vi "Autonomous Independent.vi"() -> ()   [LabVIEW 2017]
doc: "This VI is called when autonomous begins, and will automatically be terminated when autonomous ends. You can carry out timed or sensor driven robot movement independently without needing to return to the caller."
uses:
  <vilib>/Rock Robotics/WPI/Utilities/WPI_GetSetVariantRefNum.vi
  <vilib>/Rock Robotics/Network Tables/NT Read String.vi
  <vilib>/Rock Robotics/WPI/RobotDrive/WPI_RobotDriveArcadeDrive_Standard(NoSaturation).vi
  <vilib>/Rock Robotics/Network Tables/NT Write Numeric Array.vi
panel:
  out "Current Movement, for debugging":T1 {"Y Joystick Value" scale=1.0..-1.0; "X Joystick Value" scale=-1.0..1.0}
  in  "Array of robot movements":T2(array[cluster])=[{"X Joystick Value"=0.39393939393939403, "Y Joystick Value"=0.0, "Delay (sec)"=1.0, "Movement Name"="turn"}, {"X Joystick Value"=-0.3737373737373737, "Y Joystick Value"=0.0, "Delay (sec)"=1.0, "Movement Name"="turn back"}] {"Y Joystick Value" scale=1.0..-1.0; "X Joystick Value" scale=-1.0..1.0}
  # "Be sure to right-click and choose Data Operations>>Make Current Value default if you want to save the array values with the VI"
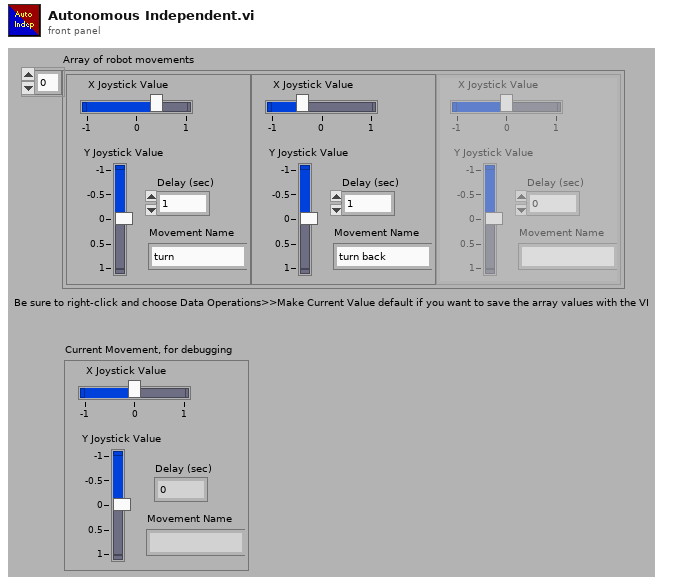
[diagram p1: front panel]
types:
  T1 = cluster{"X Joystick Value":dbl, "Y Joystick Value":dbl, "Delay (sec)":dbl, "Movement Name":string}
  T2 = cluster{"X Joystick Value":dbl, "Y Joystick Value":dbl, "Delay (sec)":dbl, "Movement Name":string}[]
  T3 = typedef "WPI_JoystickDevRef.ctl" = cluster{"Device":T4}
  T4 = typedef "WPI_JoystickDeviceEnum.ctl" = enum16{"USB 0", "USB 1", "USB 2", "USB 3", "USB 4", "USB 5"}
  T5 = typedef "WPI_RobotDriveDevRef.ctl" = cluster{"DevStatus":errorcluster, "Motors[]":T6[], "Square Inputs":bool, "Max Output":dbl}
  T6 = typedef "WPI_MotorControlDeviceRef.ctl" = cluster{"DeviceStatus":errorcluster, "Type":T7, "PWM":cluster{"PWM Channel":T8, "DeadBand":T9}, "CAN":cluster{"Device Number":u8, "SetOutput VI Ref":variant, "GetOutput VI Ref":variant, "Enable VI Ref":variant, "Disable VI Ref":variant, "Data":variant}, "Invert":bool, "DIO PWM":cluster{"PWM \"Enable\" Channel":T8, "DIOChannel":T10, "PWM Rate":dbl}}
  T7 = typedef "WPI_MotorControlType.ctl" = enum16{"PWM", "CAN", "DIO PWM"}
  T8 = typedef "FPGA_DIOPWMChannel.ctl" = enum8{"PWM 0", "PWM 1", "PWM 2", "PWM 3", "PWM 4", "PWM 5", "PWM 6", "PWM 7", "PWM 8", "PWM 9", "PWM MXP 0", "PWM MXP 1", "PWM MXP 2", "PWM MXP 3", "PWM MXP 4", "PWM MXP 5", "PWM MXP 6", "PWM MXP 7", "PWM MXP 8", "PWM MXP 9", "Invalid"}
  T9 = typedef "WPI_PWMDeadband.ctl" = cluster{"Name":string, "maxPositivePwm":i32, "minPositivePwm":i32, "centerPwm":i32, "maxNegativePwm":i32, "minNegativePwm":i32, "angularRange":u16}
  T10 = typedef "FPGA_DIOChannel.ctl" = enum8{"DIO 0", "DIO 1", "DIO 2", "DIO 3", "DIO 4", "DIO 5", "DIO 6", "DIO 7", "DIO 8", "DIO 9", "DIO MXP 0", "DIO MXP 1", "DIO MXP 2", "DIO MXP 3", "DIO MXP 4", "DIO MXP 5", "DIO MXP 6", "DIO MXP 7", "DIO MXP 8", "DIO MXP 9", "DIO MXP 10", "DIO MXP 11", "DIO MXP 12", "DIO MXP 13", "DIO MXP 14", "DIO MXP 15", "SPI Port CS1", "SPI Port CS2", "SPI Port CS3", "SPI Port MISO", "SPI Port MOSI", "Invalid"}
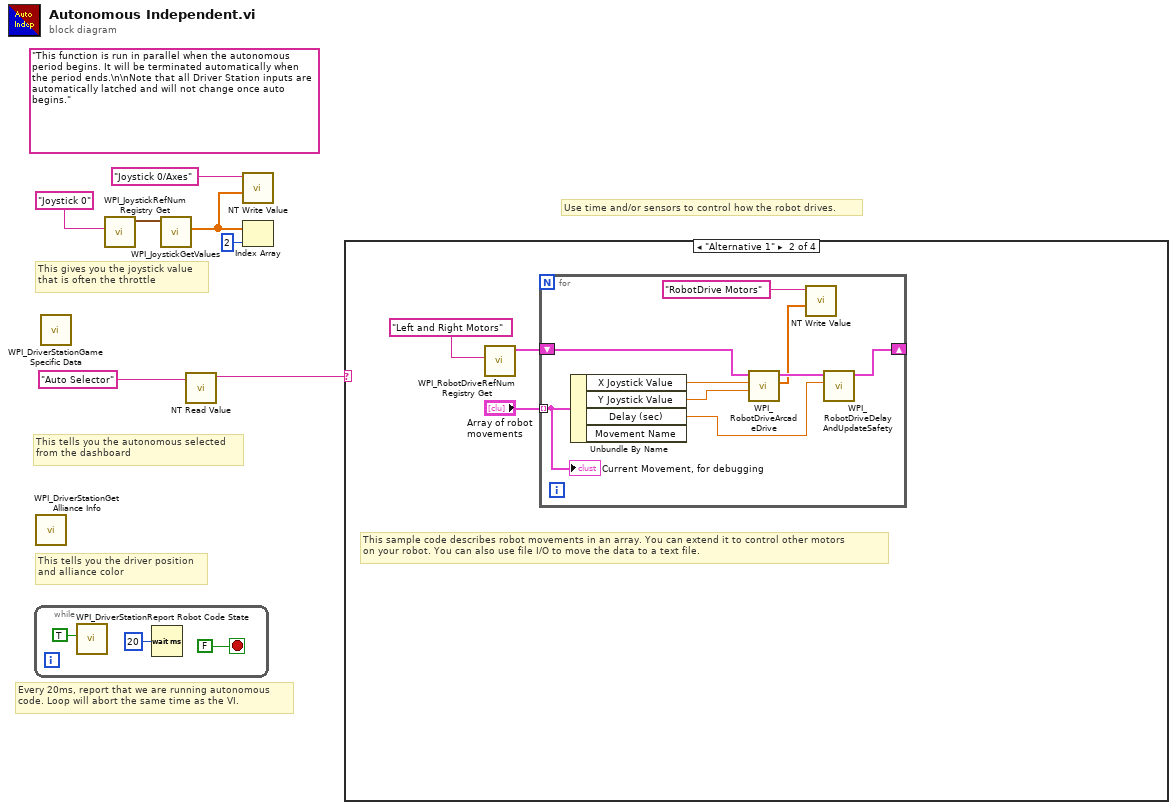
[diagram p0: block diagram]
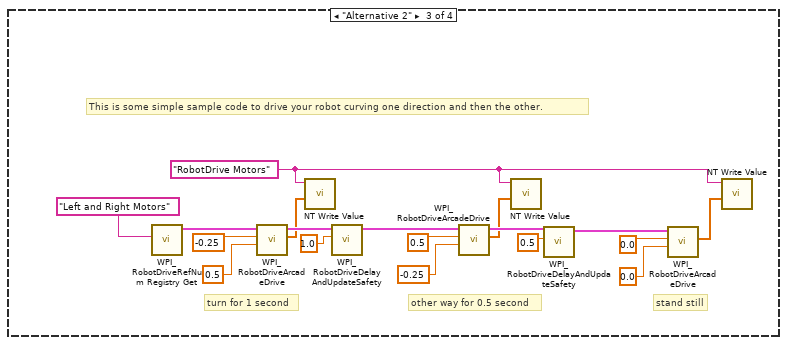
[diagram p3: hidden frame]
diagram:
  (unwired) "This function is run in parallel when the autonomous period begins. It will be terminated automatically when the period ends.\n\nNote that all Driver Station inputs are automatically latched and will not change once auto begins."
  # "This tells you the autonomous selected\nfrom the dashboard"
  # "Every 20ms, report that we are running autonomous\ncode. Loop will abort the same time as the VI."
  # "This gives you the joystick value\nthat is often the throttle"
  # "Use time and/or sensors to control how the robot drives."
  # "This tells you the driver position\nand alliance color"
  n1 = while {
    stop <- FALSE stop-if-true
    n2 = call <vilib>:"WPI_DriverStationReport Robot Code State.vi"("Autonomous"=TRUE) -> ()  [unwired: 10 in, 1 out]
    n3 = Wait (ms)(milliseconds to wait=u32 20) -> ()  [unwired: 1 out]
  }
  n4 = call <vilib>:"WPI_DriverStationGet Alliance Info.vi"() -> ()  [unwired: 12 out]
  n5 = call <vilib>:"WPI_DriverStationGame Specific Data.vi"() -> ()  [unwired: 11 in, 1 out]
  n6 = call <vilib>:"WPI_JoystickRefNum Registry Get.vi"("refnum name"="Joystick 0") -> ("JoystickDevRef"=w6:T3)  [unwired: 1 in, 9 out]
  n7 = call <vilib>:"WPI_JoystickGetValues.vi"("JoystickDevRef"=w6) -> ("Axes"=w2:dbl[])  [unwired: 6 in, 4 out]
  n8 = call-poly <vilib>:"NT Read Value.vi"("Name"="Auto Selector") -> ("String"=w3:string)  [unwired: 9 in, 1 out]
  n9 = call-poly <vilib>:"NT Write Value.vi"("Numeric Array"=w2, "Name"="Joystick 0/Axes") -> ()  [unwired: 9 in, 1 out]
  n10 = Index Array(array=w2, index=2) -> ()  [unwired: 1 out]
  n11 = case shown="\"Alternative 1\"" w3 {
    frame Default {
      # "You can put your main auto here, or you can right-click on the case and make any\nother frame be the default case."
      # "This is the frame that will execute if no selection is made, or if it is not recognized"
    }
    frame "Alternative 1" {
      # "This sample code describes robot movements in an array. You can extend it to control other motors\non your robot. You can also use file I/O to move the data to a text file."
      n12 = call <vilib>:"WPI_RobotDriveRefNum Registry Get.vi"("refnum name"="Left and Right Motors") -> ("RobotDriveDevRef"=w12:T5)  [unwired: 1 in, 9 out]
      n13 = for {
        shift-right: [w20] -> _
        shift-left: w12 -> [w21]
        tunnel: "Array of robot movements" -> [w16] mode=indexing
        n14 = Unbundle By Name(w16) -> ("X Joystick Value"=w19:dbl, "Y Joystick Value"=w18:dbl, "Delay (sec)"=w17:dbl)  [unwired: 1 out]
        n15 = call-poly <vilib>:"WPI_RobotDriveArcadeDrive.vi"("Y axis value"=w18, "X axis value"=w19, "RobotDriveDevRef"=w21) -> ("Motor Values"=w14:dbl[], "RobotDriveDevRef"=w22:T5)  [unwired: 1 in, 6 out]
        n16 = call-poly <vilib>:"NT Write Value.vi"("Numeric Array"=w14, "Name"="RobotDrive Motors") -> ()  [unwired: 9 in, 1 out]
        n17 = call <vilib>:"WPI_RobotDriveDelayAndUpdateSafety.vi"("Delay (s)"=w17, "RobotDriveDevRef"=w22) -> ("RobotDriveDevRef 2"=w20:T5)  [unwired: 8 in, 1 out]
        "Current Movement, for debugging" <- w16
      }
    }
    frame "Alternative 2" {
      w24 = "RobotDrive Motors" ("Name")
      # "This is some simple sample code to drive your robot curving one direction and then the other."
      # "stand still"
      # "other way for 0.5 second"
      # "turn for 1 second"
      n18 = call <vilib>:"WPI_RobotDriveRefNum Registry Get.vi"("refnum name"="Left and Right Motors") -> ("RobotDriveDevRef"=w40:T5)  [unwired: 1 in, 9 out]
      n19 = call-poly <vilib>:"WPI_RobotDriveArcadeDrive.vi"("Y axis value"=0.5 ("X axis value"), "X axis value"=-0.25, "RobotDriveDevRef"=w40) -> ("Motor Values"=w23:dbl[], "RobotDriveDevRef"=w33:T5)  [unwired: 1 in, 6 out]
      n20 = call-poly <vilib>:"NT Write Value.vi"("Numeric Array"=w23, "Name"=w24) -> ()  [unwired: 9 in, 1 out]
      n21 = call <vilib>:"WPI_RobotDriveDelayAndUpdateSafety.vi"("Delay (s)"=1.0, "RobotDriveDevRef"=w33) -> ("RobotDriveDevRef 2"=w34:T5)  [unwired: 8 in, 1 out]
      n22 = call-poly <vilib>:"WPI_RobotDriveArcadeDrive.vi"("Y axis value"=-0.25 ("X axis value"), "X axis value"=0.5, "RobotDriveDevRef"=w34) -> ("Motor Values"=w25:dbl[], "RobotDriveDevRef"=w35:T5)  [unwired: 1 in, 6 out]
      n23 = call-poly <vilib>:"NT Write Value.vi"("Numeric Array"=w25, "Name"=w24) -> ()  [unwired: 9 in, 1 out]
      n24 = call <vilib>:"WPI_RobotDriveDelayAndUpdateSafety.vi"("Delay (s)"=0.5, "RobotDriveDevRef"=w35) -> ("RobotDriveDevRef 2"=w36:T5)  [unwired: 8 in, 1 out]
      n25 = call-poly <vilib>:"WPI_RobotDriveArcadeDrive.vi"("Y axis value"=0.0 ("X axis value"), "X axis value"=0.0, "RobotDriveDevRef"=w36) -> ("Motor Values"=w26:dbl[])  [unwired: 1 in, 7 out]
      n26 = call-poly <vilib>:"NT Write Value.vi"("Numeric Array"=w26, "Name"=w24) -> ()  [unwired: 9 in, 1 out]
    }
    frame "Your Turn" {
    }
  }
